vi "WriteRaisedAlarms.vi"(8 "ErrorIn":errorcluster, 10 "RaisedAlarms":refnum<class "IAlarm.lvclass">[](array[class]), 11 "IResultIn":refnum<class "IResult.lvclass">) -> (0 "ErrorOut":errorcluster, 3 "IResultOut":refnum<class "IResult.lvclass">)   [LabVIEW 2019]
uses:
  IResult.lvclass
  Alarm/IAlarm.lvclass
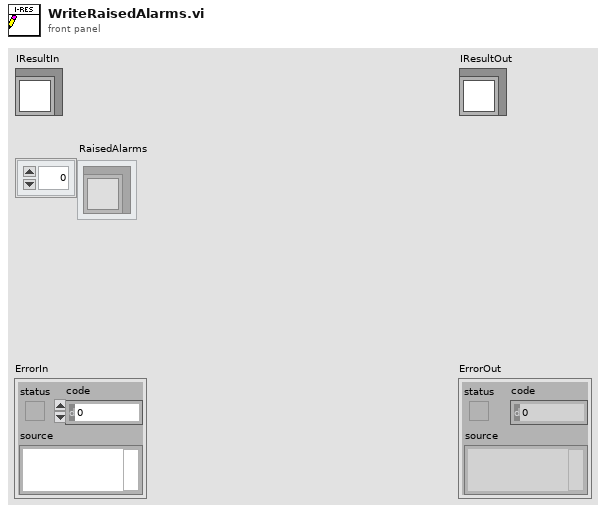
[diagram p1: front panel]
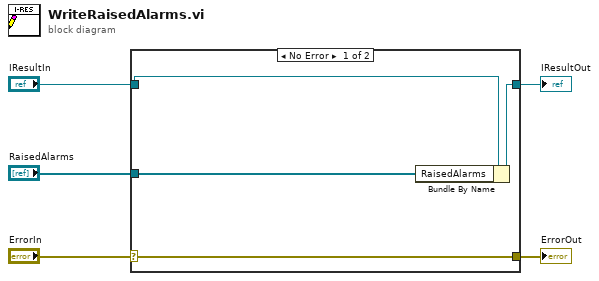
[diagram p0: block diagram]
diagram:
  n1 = case shown="No Error" "ErrorIn" {
    selector: "ErrorIn" -> [w9 w10]
    tunnel: [w9 w10] -> w4
    tunnel: [w7 w11] -> w2
    tunnel: "IResultIn" -> [w8 w11]
    tunnel: "RaisedAlarms" -> [w6 _]
    frame No Error {
      n2 = Bundle By Name(cluster=w8, "RaisedAlarms"=w6) -> (w7:refnum<class "IResult.lvclass">)
    }
    frame Error {
    }
  }
  "ErrorOut" <- w4
  "IResultOut" <- w2
